vi "LLXPC 71-146 TCP BACKEND AMP2.vi"() -> ()   [LabVIEW 2013]
uses:
  shared/stop FGV control.ctl
  LLXPC 71-146 TCP BE Stat AMP2.vi
panel:
  in  "remote port or service name":u16=2440
  out "Read_Error":errorcluster
  out "output cluster":T1={"Result"=6.15, "Result"=6.15, "Result"=20.8, "Result"=21.3}
  out "mseconds":dbl
  out "Read_Q_Error":errorcluster
  out "State":i32=4
  in  "state time":u32=200
  in  "stop":bool
  out "Open Status Connection":errorcluster
  in  "Source_URL":string="192.168.13.98"
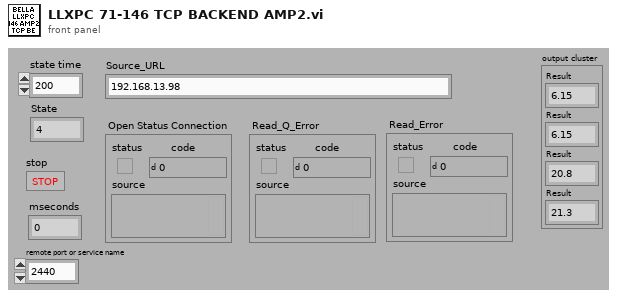
[diagram p1: front panel]
types:
  T1 = cluster{"Result":dbl, "Result":dbl, "Result":dbl, "Result":dbl}
  T2 = cluster{bool, bool, bool, bool, bool, bool, bool, bool, bool, bool, bool, bool, bool, bool, bool, bool}
  T3 = cluster{cluster{bool, bool, bool, bool, bool, bool, bool, bool, bool, bool, bool, bool, bool, bool, bool, bool}, cluster{bool, bool, bool, bool, bool, bool, bool, bool, bool, bool, bool, bool, bool, bool, bool, bool}, cluster{bool, bool, bool, bool, bool, bool, bool, bool, bool, bool, bool, bool, bool, bool, bool, bool}, cluster{bool, bool, bool, bool, bool, bool, bool, bool, bool, bool, bool, bool, bool, bool, bool, bool}}
  T4 = cluster{cluster{cluster{bool, bool, bool, bool, bool, bool, bool, bool, bool, bool, bool, bool, bool, bool, bool, bool}, cluster{bool, bool, bool, bool, bool, bool, bool, bool, bool, bool, bool, bool, bool, bool, bool, bool}, cluster{bool, bool, bool, bool, bool, bool, bool, bool, bool, bool, bool, bool, bool, bool, bool, bool}, cluster{bool, bool, bool, bool, bool, bool, bool, bool, bool, bool, bool, bool, bool, bool, bool, bool}}, dbl, "output cluster":cluster{"Result":dbl, "Result":dbl, "Result":dbl, "Result":dbl}, bool, "connection ID out":refnum<k5>, "connection ID out":refnum<k5>}
  T5 = typedef "stop FGV control.ctl" = enum16{"Clear", "Write", "Read"}
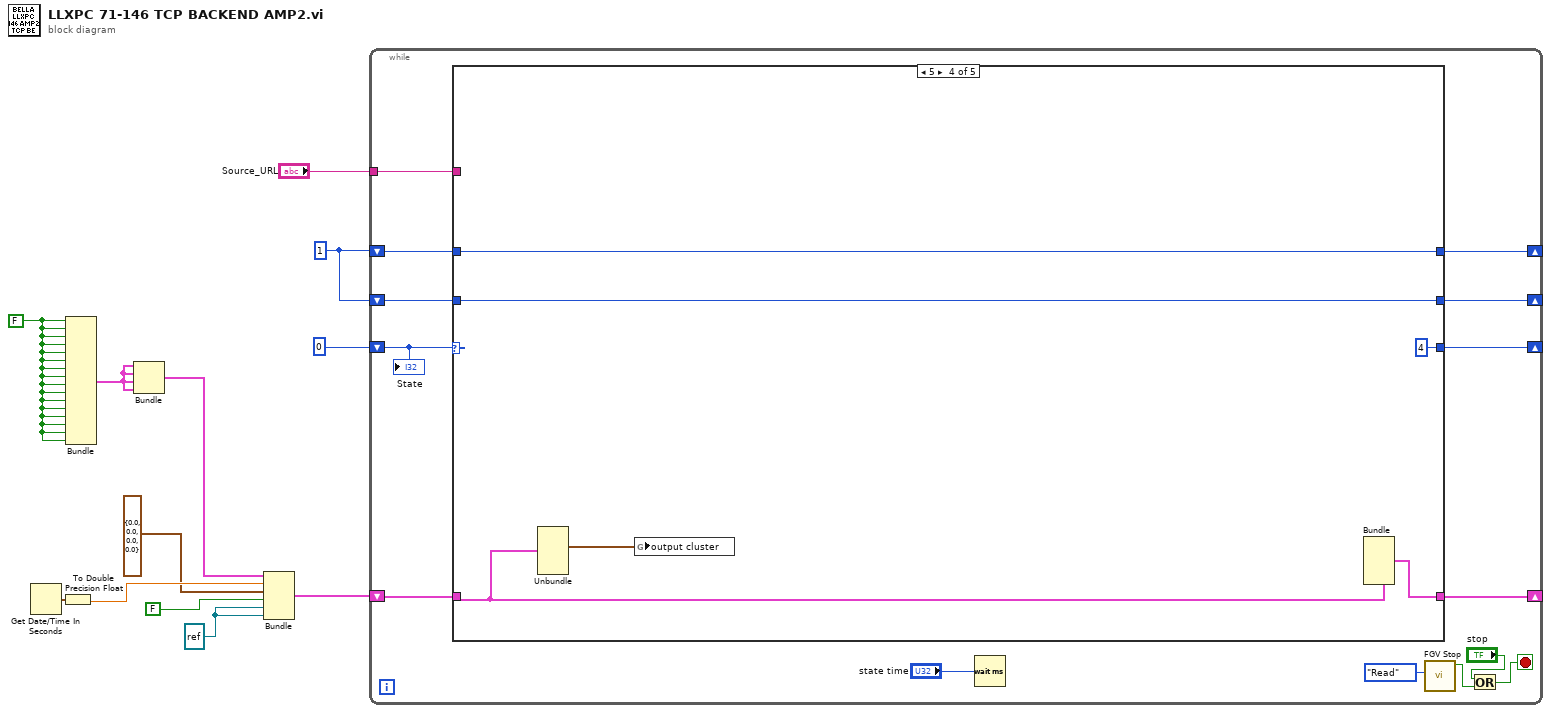
[diagram p0: block diagram]
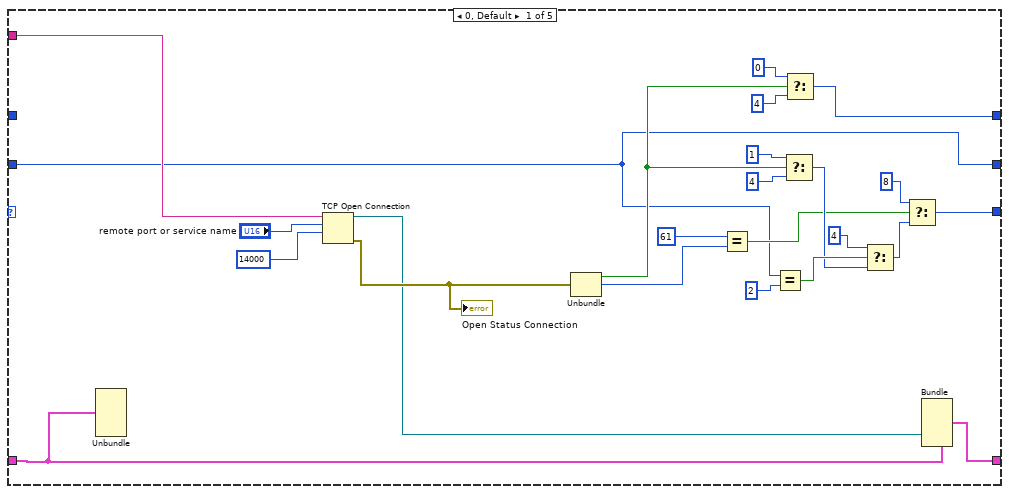
[diagram p2: hidden frame]
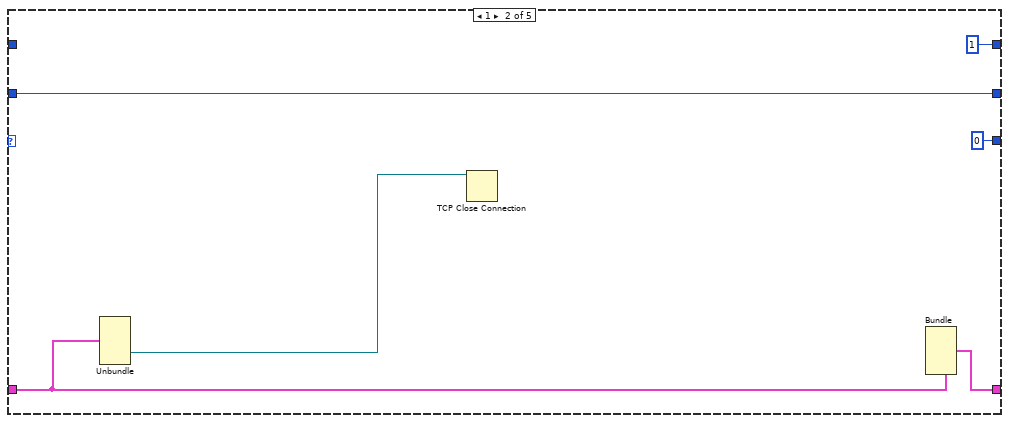
[diagram p3: hidden frame]
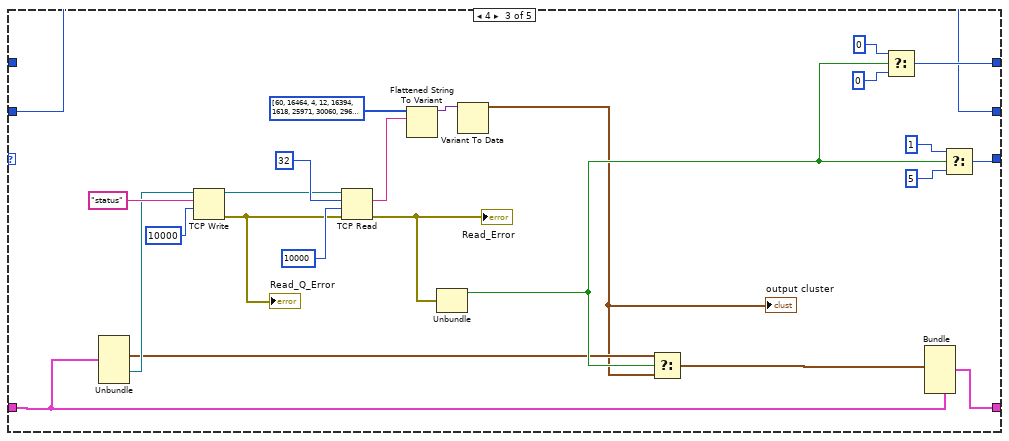
[diagram p4: hidden frame]
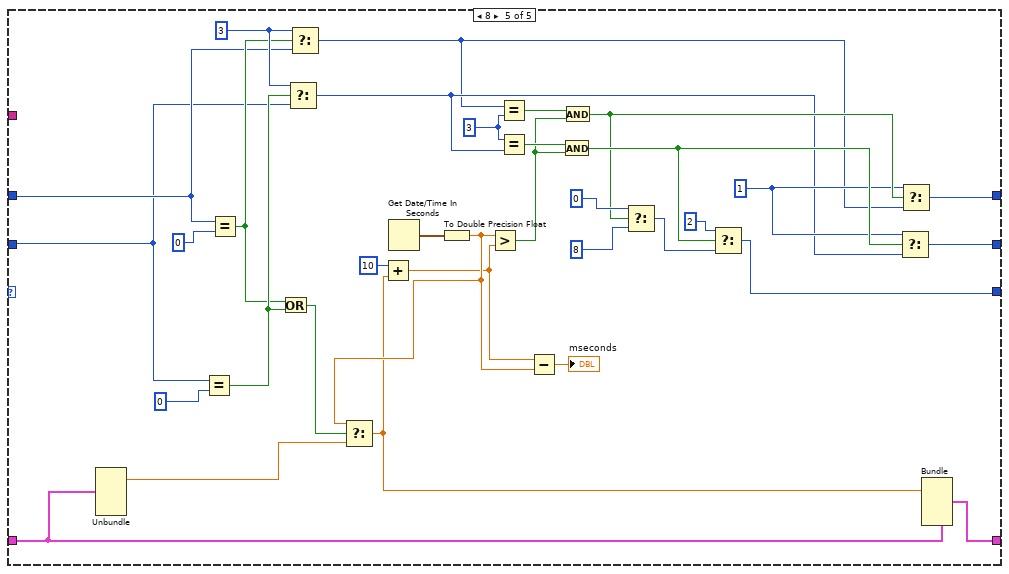
[diagram p5: hidden frame]
diagram:
  w2 = 1
  w9 = refnum<k5> refnum ("connection ID out")
  w12 = FALSE
  n1 = Get Date/Time In Seconds() -> (seconds since 1Jan1904=w10:timestamp)
  n2 = To Double Precision Float(number=w10) -> (double precision float=w7:dbl)
  n3 = Bundle(w12, w12, w12, w12, w12, w12, w12, w12, w12, w12, w12, w12, w12, w12, w12, w12) -> (w11:T2)  [unwired: 1 in]
  n4 = Bundle(w11, w11, w11, w11) -> (w6:T3)  [unwired: 1 in]
  n5 = Bundle(w6, w7, "output cluster"=T1 {"Result"=0.0, "Result"=0.0, "Result"=0.0, "Result"=0.0}, FALSE, "connection ID out"=w9, "connection ID out"=w9) -> (w5:T4)  [unwired: 1 in]
  n6 = while {
    shift-right: [w24] -> _
    shift-left: w5 -> [w25]
    shift-right: [w23] -> _
    shift-left: 0 -> [w26]
    tunnel: "Source_URL" -> [w22]
    shift-right: [w19] -> _
    shift-left: w2 -> [w20]
    shift-right: [w18] -> _
    shift-left: w2 -> [w17]
    stop <- w13 stop-if-true
    n7 = case shown="5" w26 {
      tunnel: w25 -> [w50 w56 w80 w86 w119]
      tunnel: [w49 w55 w79 w85 w118] -> w24
      tunnel: [w31 0 ("f") w70 4 ("f") w89] -> w23
      tunnel: w22 -> [w44 _ _ _ _]
      tunnel: w20 -> [w27 w51 w68 w82 w92]
      tunnel: [w27 w51 w68 w82 w90] -> w19
      tunnel: [w28 1 ("t") w69 w83 w91] -> w18
      tunnel: w17 -> [_ _ _ w83 w93]
      frame 0, Default {
        n8 = Unbundle(w50) -> ()  [unwired: 6 out]
        n9 = TCP Open Connection(address=w44, remote port or service name="remote port or service name", timeout ms (60000)=14000 ("ms timeout (10000)")) -> (connection ID=w45:refnum<k5>, error out=w46:errorcluster)  [unwired: 2 in]
        "Open Status Connection" <- w46
        n10 = Unbundle(w46) -> ("status"=w30:bool, "code"=w29:i32)  [unwired: 1 out]
        n11 = Equal?(x=61, y=w29) -> (x = y?=w36:bool)
        n12 = Equal?(x=w27, y=2 ("x")) -> (x = y?=w40:bool)
        n13 = Select(t=1, s=w30, f=4) -> (s? t:f=w39:i32)
        n14 = Select(t=0, s=w30, f=4) -> (s? t:f=w28:i32)
        n15 = Select(t=4 ("x"), s=w40, f=w39) -> (s? t:f=w37:i32)
        n16 = Select(t=8, s=w36, f=w37) -> (s? t:f=w31:i32)
        n17 = Bundle(cluster=w50, "connection ID out"=w45) -> (w49:T4)  [unwired: 5 in]
      }
      frame 1 {
        n18 = Unbundle(w56) -> ("connection ID out"=w54:refnum<k5>)  [unwired: 5 out]
        n19 = TCP Close Connection(connection ID=w54) -> ()  [unwired: 2 in, 2 out]
        n20 = Bundle(cluster=w56) -> (w55:T4)  [unwired: 6 in]
      }
      frame 4 {
        n21 = Unbundle(w80) -> ("output cluster"=w66:T1, "connection ID out"=w76:refnum<k5>)  [unwired: 4 out]
        n22 = TCP Write(connection ID=w76, data in="status", 9:10000 ("timeout ms (25000)")) -> (connection ID out=w60:refnum<k5>, error out=w59:errorcluster)  [unwired: 1 in, 1 out]
        "Read_Q_Error" <- w59
        n23 = TCP Read(connection ID=w60, bytes to read=32 ("length"), error in (no error)=w59, 9:10000 ("ms timeout (10000)")) -> (data out=w64:string, error out=w58:errorcluster)  [unwired: 1 in, 1 out]
        "Read_Error" <- w58
        n24 = Flattened String To Variant(6:w64, 7:i16[] [60, 16464, 4, 12, 16394, 1618, 25971, 30060, 29696, 12, 16394, 1618, 25971, 30060, 29696, 12, 16394, 1618, 25971, 30060, 29696, 12, 16394, 1618, 25971, 30060, 29696, 1092, 16724, 16640] ("type string")) -> (3:w63:variant)  [unwired: 1 in, 1 out]
        n25 = Unbundle(w58) -> ("status"=w71:bool)  [unwired: 2 out]
        n26 = Variant To Data(Variant=w63) -> (data=w57:T1)  [unwired: 2 in, 1 out]
        "output cluster" <- w57
        n27 = Select(t=w66, s=w71, f=w57) -> (s? t:f=w67:T1)
        n28 = Select(t=0, s=w71, f=0) -> (s? t:f=w69:i32)
        n29 = Bundle(cluster=w80, "output cluster"=w67) -> (w79:T4)  [unwired: 5 in]
        n30 = Select(t=1, s=w71, f=5) -> (s? t:f=w70:i32)
      }
      frame 5 {
        n31 = Unbundle(w86) -> ("output cluster"=w81:T1)  [unwired: 5 out]
        n32 = global write "LLXPC 71-146 TCP BE Stat AMP2.vi" "output cluster"(w81) -> ()
        n33 = Bundle(cluster=w86) -> (w85:T4)  [unwired: 6 in]
      }
      frame 8 {
        w104 = 3
        w101 = 3
        w108 = 1 ("f")
        n34 = Unbundle(w119) -> (w88:dbl)  [unwired: 5 out]
        n35 = Equal?(x=w92, y=0) -> (x = y?=w100:bool)
        n36 = Equal?(x=w93, y=0) -> (x = y?=w99:bool)
        n37 = Or(x=w99, y=w100) -> (x .or. y?=w98:bool)
        n38 = Select(t=w101, s=w100, f=w92) -> (s? t:f=w103:i32)
        n39 = Select(t=w101, s=w99, f=w93) -> (s? t:f=w102:i32)
        n40 = Get Date/Time In Seconds() -> (seconds since 1Jan1904=w95:timestamp)
        n41 = To Double Precision Float(number=w95) -> (double precision float=w117:dbl)
        n42 = Select(t=w117, s=w98, f=w88) -> (s? t:f=w87:dbl)
        n43 = Add(x=10, y=w87) -> (x+y=w116:dbl)
        n44 = Greater?(x=w117, y=w116) -> (0:w106:bool)
        n45 = Equal?(x=w102, y=w104) -> (x = y?=w105:bool)
        n46 = Equal?(x=w104, y=w103) -> (x = y?=w107:bool)
        n47 = Subtract(x=w116, y=w117) -> (x-y=→"mseconds":dbl)
        n48 = And(x=w107, y=w106) -> (x .and. y?=w113:bool)
        n49 = And(x=w105, y=w106) -> (x .and. y?=w109:bool)
        n50 = Select(t=0, s=w109, f=8) -> (s? t:f=w112:i32)
        n51 = Select(t=2, s=w113, f=w112) -> (s? t:f=w89:i32)
        n52 = Select(t=w108, s=w113, f=w103) -> (s? t:f=w90:i32)
        n53 = Select(t=w108, s=w109, f=w102) -> (s? t:f=w91:i32)
        n54 = Bundle(cluster=w119, w87) -> (w118:T4)  [unwired: 5 in]
      }
    }
    n55 = Wait (ms)(milliseconds to wait="state time") -> ()  [unwired: 1 out]
    n56 = call "FGV Stop.vi"("Function"=stop_FGV_control."Read") -> ("stop out"=w14:bool)  [unwired: 9 in, 1 out]
    n57 = Or(x="stop", y=w14) -> (x .or. y?=w13:bool)
    "State" <- w26
  }
